vi "enCOB-ID.vi"(1 "Function code":T1 items=["NMT", "SYNC", "TIME STAMP", "EMERGENCY", "PDO1 (tx)", "PDO1 (rx)", "PDO2 (tx)", "PDO2 (rx)", "PDO3 (tx)", "PDO3 (rx)", "PDO4 (tx)", "PDO4 (rx)", "SDO (tx)", "SDO (rx)", "NMT Error Control"], 2 "Node ID":u8) -> (0 "Cob ID":u32)   [LabVIEW 2023, in "canopen.lvlib" / "CANopen.lvclass"]
doc: "Computes the canonical COB-ID given the function code and the node ID. The implementation follows the algorithm described in CiA draft standard 301, page 78."
uses:
  CANopen.lvclass
  FunctionCode.ctl
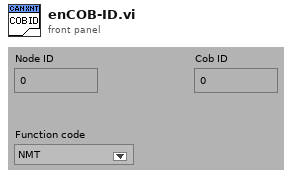
[diagram p1: front panel]
types:
  T1 = typedef "canopen.lvlib/CANopen.lvclass/FunctionCode.ctl" = u8
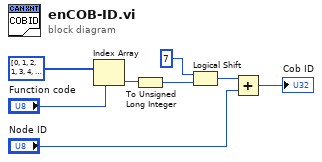
[diagram p0: block diagram]
diagram:
  n1 = Index Array(array=u8[] [0, 1, 2, 1, 3, 4, 5, 6, 7, 8, 9, 10, 11, 12, 14], index="Function code") -> (element=w5:u8)
  n2 = To Unsigned Long Integer(number=w5) -> (unsigned 32bit integer=w4:u32)
  n3 = Logical Shift(y=i16 7, x=w4) -> (x << y=w3:u32)
  n4 = Add(x=w3, y="Node ID") -> (x+y=→"Cob ID":u32)
